vi "Fetch Waveform Measurement.vi"(6 "Maximum Time (10000 ms)":u32=10000, 7 "Measurement Function (0: Rise Time)":u16(ring) items=["Rise Time", "Fall Time", "Frequency", "Duty Cycle Negative", "Duty Cycle Positive", "Width Negative", "Width Positive", "Over Shoot", "Pre Shoot", "Period", "Amplitude", "Voltage Average", "Voltage Base", "Voltage Max", "Voltage Min", "Voltage Vpp", "Voltage RMS", "Voltage Top", "Phase Negative", "Phase Positive", "Delay Negative", "Delay Positive"], 8 "error in (no error)":errorcluster, 9 "Source Channel 2 (2: Channel 2)":u16(ring)=2 items=["Channel 1"=1, "Channel 2"=2, "Channel 3"=3, "Channel 4"=4], 10 "Source Channel (1: Channel 1)":u16(ring)=1 items=["Channel 1"=1, "Channel 2"=2, "Channel 3"=3, "Channel 4"=4], 11 "VISA resource name":refnum<visa-resource-name>) -> (0 "error out":errorcluster, 2 "Measurement":dbl, 3 "VISA resource name out":refnum<visa-resource-name>)   [LabVIEW 2010, in "Agilent DSO1000 Series.lvlib"]
doc: "Obtains a waveform measurement and returns the measurement value. You specify a particular measurement type, such as rise time, frequency, and voltage peak-to-peak. The waveform on which the oscilloscope calculates the waveform measurement is from an acquisition that you previously initiated. \n\nYou call this VI separately for each waveform measurement you want to obtain on a specific channel.\n\n<B>Notes:</B>\n\n(1) You must configure the appropriate reference levels before you call this VI to take a rise time, fall time, width negative, width positive, duty cycle negative, or duty cycle positive measurement.\n\n(2) This VI does not check the instrument status. Typically, you call this VI only in a sequence of calls to other low-level driver VIs. The sequence performs one operation. You use the low-level VIs to optimize one or more aspects of interaction with the instrument."
uses:
  <instrlib>/Agilent DSO1000 Series/Agilent DSO1000 Series.lvlib
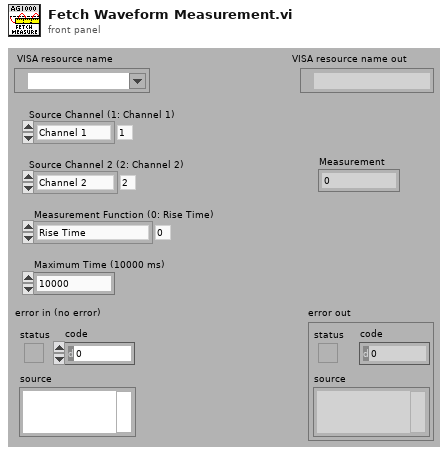
[diagram p1: front panel]
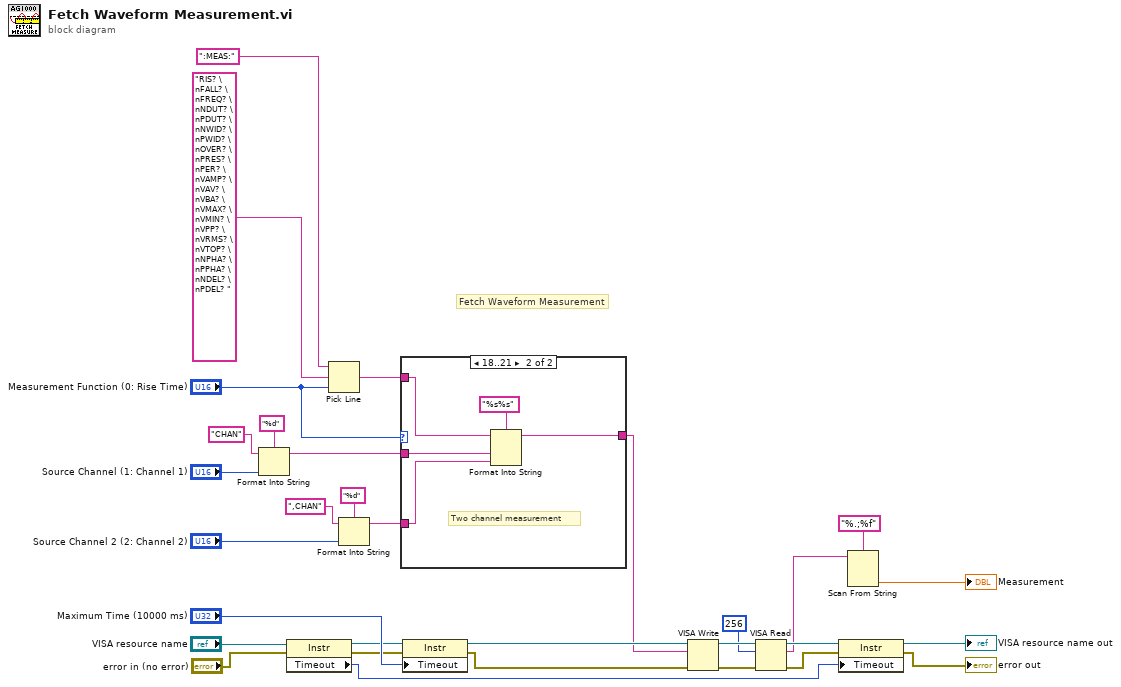
[diagram p0: block diagram]
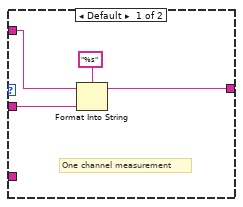
[diagram p2: hidden frame]
diagram:
  # "Fetch Waveform Measurement"
  n1 = Format Into String(format string="%d", initial string="CHAN" ("multi-line string"), "Source Channel (1: Channel 1)") -> (resulting string=w4:string)  [unwired: 1 in, 1 out]
  n2 = property class="Instr"(reference="VISA resource name", error in="error in (no error)") -> (reference out=w27:refnum<visa-resource-name>, error out=w28:errorcluster, "Timeout"=w13:u32)
  n3 = Pick Line(string ("")=":MEAS:", multi-line string="RIS? \nFALL? \nFREQ? \nNDUT? \nPDUT? \nNWID? \nPWID? \nOVER? \nPRES? \nPER? \nVAMP? \nVAV? \nVBA? \nVMAX? \nVMIN? \nVPP? \nVRMS? \nVTOP? \nNPHA? \nPPHA? \nNDEL? \nPDEL? ", line index="Measurement Function (0: Rise Time)") -> (output string=w3:string)
  n4 = Format Into String(format string="%d", initial string=",CHAN" ("multi-line string"), "Source Channel 2 (2: Channel 2)") -> (resulting string=w2:string)  [unwired: 1 in, 1 out]
  n5 = case shown="18..21" "Measurement Function (0: Rise Time)" {
    tunnel: w4 -> [w34 w38]
    tunnel: w3 -> [w35 w39]
    tunnel: [w32 w36] -> w1
    tunnel: w2 -> [_ w37]
    frame Default {
      # "One channel measurement"
      n6 = Format Into String(format string="%s", initial string=w35, w34) -> (resulting string=w32:string)  [unwired: 1 in, 1 out]
    }
    frame 18..21 {
      # "Two channel measurement"
      n7 = Format Into String(format string="%s%s", initial string=w39, w38, w37) -> (resulting string=w36:string)  [unwired: 1 in, 1 out]
    }
  }
  n8 = property class="Instr"(reference=w27, error in=w28, "Timeout"="Maximum Time (10000 ms)") -> (reference out=w18:refnum<visa-resource-name>, error out=w17:errorcluster)
  n9 = VISA Write(VISA resource name=w18, write buffer=w1, error in (no error)=w17) -> (VISA resource name out=w15:refnum<visa-resource-name>, error out=w16:errorcluster)  [unwired: 1 out]
  n10 = VISA Read(VISA resource name=w15, byte count=u32 256, error in (no error)=w16) -> (VISA resource name out=w11:refnum<visa-resource-name>, read buffer=w8:string, error out=w12:errorcluster)  [unwired: 1 out]
  n11 = property class="Instr"(reference=w11, error in=w12, "Timeout"=w13) -> (reference out=→"VISA resource name out":refnum<visa-resource-name>, error out=→"error out":errorcluster)
  n12 = Scan From String(format string="%.;%f", input string=w8) -> (output 1=→"Measurement":dbl)  [unwired: 3 in, 3 out]
